vi "Get Enum Definition Details.vi"(8 "error in":errorcluster, 11 "Doc Ref":refnum<k20>) -> (0 "error out":errorcluster, 2 "Enum Definition Details":T1(array[cluster]))   [LabVIEW 2026]
uses:
  Types/NodeFilteringOptions.ctl
  <resource>/objmgr/DOMUserDefRef.rc
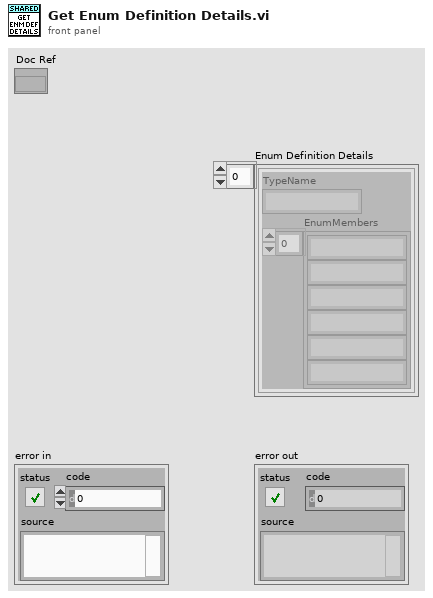
[diagram p1: front panel]
types:
  T1 = cluster{"TypeName":string, "EnumMembers":string[]}[]
  T2 = typedef "NodeFilteringOptions.ctl" = enum16{"GetCustomDeviceNode", "GetAllChannelNodes", "GetAllSectionNodes", "GetAllWaveformNodes", "GetFirstChannelNode", "GetFirstSectionNode", "GetFirstWaveformNode", "GetSpecificSectionNode", "GetSpecificCustomDeviceNode", "GetSpecificChannelNode", "GetSpecificWaveformNode", "GetMatchedNamedNode", "GetEnumDefinitionsNode", "GetSpecificEnumDefinitionNode", "GetAllEnumDefinitionNodes", "GetDynamicChannelNodes"}
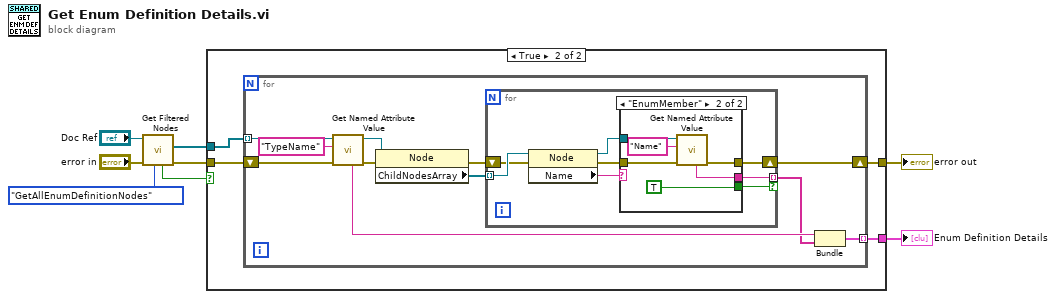
[diagram p0: block diagram]
diagram:
  n1 = call "Get Filtered Nodes.vi"("Node Filtering"=NodeFilteringOptions."GetAllEnumDefinitionNodes", "error in"="error in", "Document in"="Doc Ref") -> ("error out"=w4:errorcluster, "Filtered Nodes"=w5:refnum<k20>[], "Node Found?"=w6:bool)  [unwired: 4 in, 2 out]
  n2 = case shown="True" w6 {
    tunnel: w5 -> [_ w13]
    tunnel: w4 -> [w9 w12]
    tunnel: [_ w11] -> w3
    tunnel: [w9 w10] -> w1
    frame False {
    }
    frame True {
      n3 = for {
        tunnel: w13 -> [w24] mode=indexing
        shift-right: [w17] -> w10
        shift-left: w12 -> [w23]
        tunnel: [w14] -> w11 mode=indexing
        n4 = call "Get Named Attribute Value.vi"("error in"=w23, "Attribute Name"="TypeName", "Node In"=w24) -> ("error out"=w20:errorcluster, "Node Out"=w21:refnum<k20>, "Attribute Value"=w16:string)  [unwired: 5 in, 1 out]
        n5 = property class="Node"(reference=w21, error in=w20) -> (error out=w18:errorcluster, "ChildNodesArray"=w19:refnum<k20>[])  [unwired: 1 out]
        n6 = for {
          tunnel: w19 -> [w32] mode=indexing
          shift-right: [w27] -> w17
          shift-left: w18 -> [w31]
          tunnel: [w26] -> w15 mode=indexing if=w25
          n7 = property class="Node"(reference=w32, error in=w31) -> (reference out=w28:refnum<k20>, error out=w29:errorcluster, "Name"=w30:string)
          n8 = case shown="\"EnumMember\"" w30 {
            tunnel: w29 -> [w33 w39]
            tunnel: w28 -> [_ w38]
            tunnel: [w33 w36] -> w27
            tunnel: [_ w35] -> w26
            tunnel: [_ TRUE] -> w25
            frame "False", Default {
            }
            frame "EnumMember" {
              n9 = call "Get Named Attribute Value.vi"("error in"=w39, "Attribute Name"="Name", "Node In"=w38) -> ("error out"=w36:errorcluster, "Attribute Value"=w35:string)  [unwired: 5 in, 2 out]
            }
          }
        }
        n10 = Bundle("Attribute Value"=w16, w15) -> (w14:cluster{"Attribute Value":string, string[]})  [unwired: 1 in]
      }
    }
  }
  "Enum Definition Details" <- w3
  "error out" <- w1
